vi "SingleServiceRegistered_DiscoveryApiRoundTrip_AllNodesSucceed.vi"() -> (6 "pass":bool, 8 "result":string, 15 "error out":errorcluster)   [LabVIEW 2020]
uses:
  Runtime/Generated/Measurement Plugin Discovery Client/RPC Messages/ni_measurementlink_discovery_v1_RegisterServiceRequest.ctl
  Runtime/Generated/Measurement Plugin Discovery Client/RPC Messages/ni_measurementlink_discovery_v1_ServiceDescriptor.ctl
  Runtime/Generated/Measurement Plugin Discovery Client/RPC Messages/ni_measurementlink_discovery_v1_ServiceDescriptor_AnnotationsEntry.ctl
  Runtime/Generated/Measurement Plugin Discovery Client/RPC Messages/ni_measurementlink_discovery_v1_ServiceLocation.ctl
  Runtime/Generated/Measurement Plugin Discovery Client/RPC Messages/ni_measurementlink_discovery_v1_EnumerateServicesRequest.ctl
  Runtime/Generated/Measurement Plugin Discovery Client/RPC Messages/ni_measurementlink_discovery_v1_ResolveServiceRequest.ctl
  <vilib>/ErrorRing/Error Ring.xnode
  Runtime/Generated/Measurement Plugin Discovery Client/Measurement Plugin Discovery Client.lvlib
panel:
  out "Register assigns registration id?":bool
  out "Unregister then enumerate lists nothing?":bool
  out "Enumerate lists service?":bool
  out "Resolve matches location?":bool
  # "Test assumes discovery service has already been started."
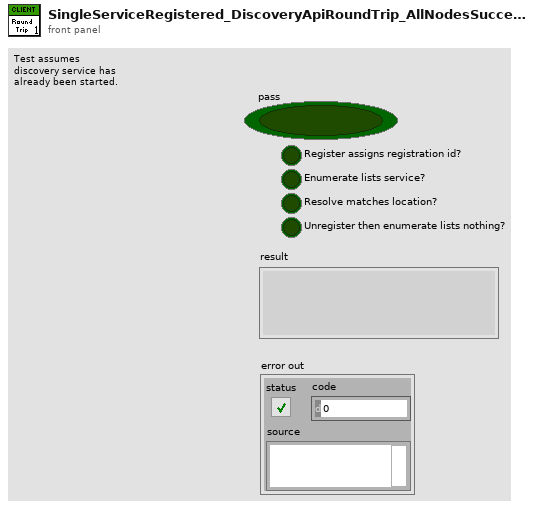
[diagram p1: front panel]
types:
  T1 = enum16{"1. Register", "2. Enumerate", "3. Resolve", "4. Unregister"}[]
  T2 = typedef "Measurement Plugin Discovery Client.lvlib/ni_measurementlink_discovery_v1_EnumerateServicesRequest.ctl" = cluster{"provided_interface":string}
  T3 = typedef "Measurement Plugin Discovery Client.lvlib/ni_measurementlink_discovery_v1_ResolveServiceRequest.ctl" = cluster{"provided_interface":string, "service_class":string}
  T4 = typedef "Measurement Plugin Discovery Client.lvlib/ni_measurementlink_discovery_v1_RegisterServiceRequest.ctl" = cluster{"service_description":T5, "location":T7}
  T5 = typedef "Measurement Plugin Discovery Client.lvlib/ni_measurementlink_discovery_v1_ServiceDescriptor.ctl" = cluster{"display_name":string, "description_url":string, "provided_interfaces":string[], "service_class":string, "annotations":T6[]}
  T6 = typedef "Measurement Plugin Discovery Client.lvlib/ni_measurementlink_discovery_v1_ServiceDescriptor_AnnotationsEntry.ctl" = cluster{"key":string, "value":string}
  T7 = typedef "Measurement Plugin Discovery Client.lvlib/ni_measurementlink_discovery_v1_ServiceLocation.ctl" = cluster{"location":string, "insecure_port":string, "ssl_authenticated_port":string}
  T8 = typedef "Measurement Plugin Discovery Client.lvlib/ni_measurementlink_discovery_v1_RegisterServiceResponse.ctl" = cluster{"registration_id":string}
  T9 = typedef "Measurement Plugin Discovery Client.lvlib/ni_measurementlink_discovery_v1_EnumerateServicesResponse.ctl" = cluster{"available_services":T5[]}
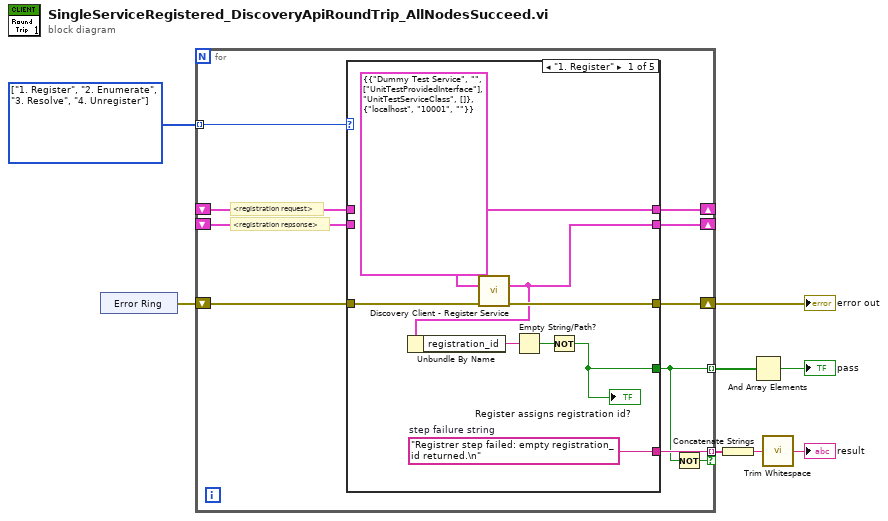
[diagram p0: block diagram]
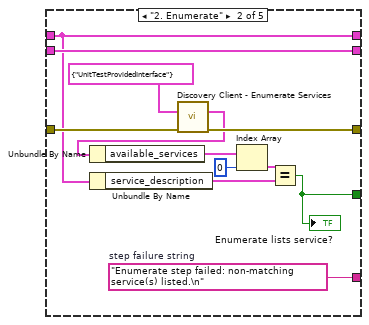
[diagram p2: hidden frame]
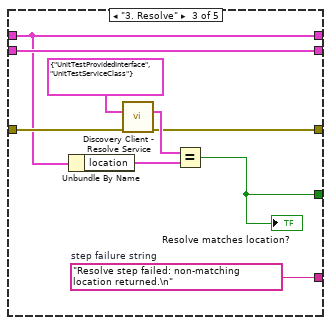
[diagram p3: hidden frame]
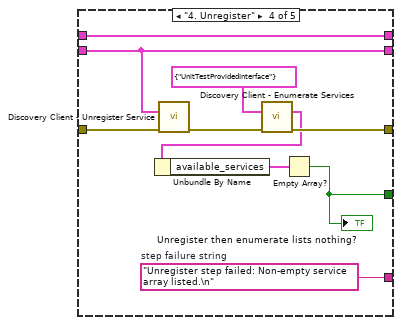
[diagram p4: hidden frame]
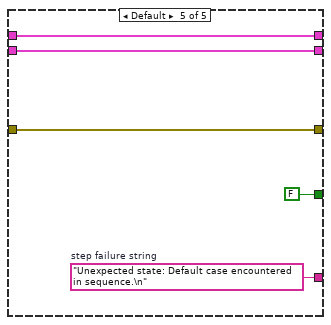
[diagram p5: hidden frame]
diagram:
  w8 = T1 [enum."1. Register", enum."2. Enumerate", enum."3. Resolve", enum."4. Unregister"] items=["1. Register", "2. Enumerate", "3. Resolve", "4. Unregister"]
  n1 = xnode "Error Ring"() -> ("error out"=w7:errorcluster)
  n2 = for {
    tunnel: w8 -> [w18] mode=indexing
    shift-right: [w16] -> w4
    shift-left: w7 -> [w17]
    shift-right: [w15] -> _
    shift-left: _ -> [w14]
    shift-right: [w13] -> _
    shift-left: _ -> [w12]
    tunnel: [w9] -> w6 mode=indexing
    tunnel: [w11] -> w2 mode=indexing if=w10
    # "<registration request>"
    # "<registration repsonse>"
    n3 = case shown="\"1. Register\"" w18 {
      tunnel: w17 -> [w26 w37 w47 w56 w62]
      tunnel: [w25 w36 w41 w53 w62] -> w16
      tunnel: [w22 w38 w46 w55 w60] -> w15
      tunnel: w14 -> [_ w38 w46 w55 w60]
      tunnel: [w19 w30 w44 w54 w59] -> w13
      tunnel: w12 -> [_ w30 w44 w54 w59]
      tunnel: [w21 w29 w42 w50 FALSE] -> w9
      tunnel: [w20 w28 w40 w49 w58] -> w11
      frame "1. Register" {
        w19 = T4 {"service_description"={"display_name"="Dummy Test Service", "description_url"="", "provided_interfaces"=["UnitTestProvidedInterface"], "service_class"="UnitTestServiceClass", "annotations"=[]}, "location"={"location"="localhost", "insecure_port"="10001", "ssl_authenticated_port"=""}} ("Request Data")
        w20 = "Registrer step failed: empty registration_id returned.\n"  # step failure string
        n4 = call "Discovery Client - Register Service.vi"("Request Data"=w19, "error in (no error)"=w26) -> ("Response Data"=w22:T8, "error out"=w25:errorcluster)  [unwired: 12 in]
        n5 = Unbundle By Name(w22) -> ("registration_id"=w23:string)
        n6 = Empty String/Path?(string/path=w23) -> (empty?=w24:bool)
        n7 = Not(x=w24) -> (.not. x?=w21:bool)
        "Register assigns registration id?" <- w21
      }
      frame "2. Enumerate" {
        w28 = "Enumerate step failed: non-matching service(s) listed.\n"  # step failure string
        n8 = Unbundle By Name(w30) -> ("service_description"=w33:T5)
        n9 = call "Discovery Client - Enumerate Services.vi"("Request Data"=T2 {"provided_interface"="UnitTestProvidedInterface"}, "error in (no error)"=w37) -> ("Response Data"=w31:T9, "error out"=w36:errorcluster)  [unwired: 12 in]
        n10 = Unbundle By Name(w31) -> ("available_services"=w34:T5[])
        n11 = Index Array(array=w34, index=0) -> (element=w35:T5)
        n12 = Equal?(x=w35, y=w33) -> (x = y?=w29:bool)
        "Enumerate lists service?" <- w29
      }
      frame "3. Resolve" {
        w40 = "Resolve step failed: non-matching location returned.\n"  # step failure string
        n13 = Unbundle By Name(w44) -> ("location"=w45:T7)
        n14 = call "Discovery Client - Resolve Service.vi"("Request Data"=T3 {"provided_interface"="UnitTestProvidedInterface", "service_class"="UnitTestServiceClass"}, "error in (no error)"=w47) -> ("Response Data"=w43:T7, "error out"=w41:errorcluster)  [unwired: 12 in]
        n15 = Equal?(x=w43, y=w45) -> (x = y?=w42:bool)
        "Resolve matches location?" <- w42
      }
      frame "4. Unregister" {
        w49 = "Unregister step failed: Non-empty service array listed.\n"  # step failure string
        n16 = call "Discovery Client - Unregister Service.vi"("Request Data"=w55, "error in (no error)"=w56) -> ("error out"=w57:errorcluster)  [unwired: 12 in, 1 out]
        n17 = call "Discovery Client - Enumerate Services.vi"("Request Data"=T2 {"provided_interface"="UnitTestProvidedInterface"}, "error in (no error)"=w57) -> ("Response Data"=w51:T9, "error out"=w53:errorcluster)  [unwired: 12 in]
        n18 = Unbundle By Name(w51) -> ("available_services"=w52:T5[])
        n19 = Empty Array?(array=w52) -> (empty?=w50:bool)
        "Unregister then enumerate lists nothing?" <- w50
      }
      frame Default {
        w58 = "Unexpected state: Default case encountered in sequence.\n"  # step failure string
      }
    }
    n20 = Not(x=w9) -> (.not. x?=w10:bool)
  }
  "error out" <- w4
  n21 = Concatenate Strings(w2) -> (w1:string)
  n22 = And Array Elements(Boolean array=w6) -> (logical AND=→"pass":bool)
  n23 = call <vilib>:"Trim Whitespace.vi"("string"=w1) -> ("trimmed string"=→"result":string)  [unwired: 1 in]
